vi "global.vi"() -> ()   [LabVIEW 2016]
panel:
  out "DATA Error":errorcluster
  out "DATA Conn":refnum<k16>
  out "CMD Error":errorcluster
  out "CMD Conn":refnum<k16>
  in  "DATA Port":u16=2048
  in  "CMD Port":u16=2047
  in  "FPGA Address":string="192.168.1.12"
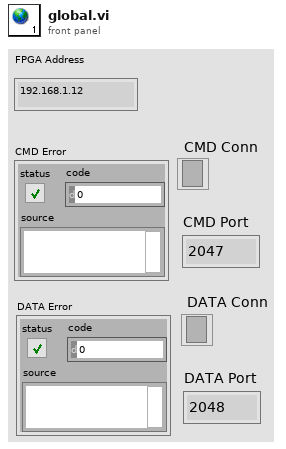
[diagram p1: front panel]
diagram:
